vi "Stop Measurement.vi"(1 "VISA resource name":refnum<visa-resource-name>="COM1", 2 "Addr (0-15)":i8 min=0 max=15 step=1) -> (0 "Stop OK":bool)   [LabVIEW 2012]
doc: "The Basic Serial Read and Write example performs a Serial Port Read, a Serial Port Write, or a combination of these actions. The user selects the actions (read or write) on the front panel. If both are selected, the VI will write the data first, read data, and then close the VISA session that is opened to the port. This VI will wait until the specified number of bytes is received at the port or until a termination character is read.\n\nINSTRUCTIONS:\n1) Select the serial resource and configuration parameters (baud rate, data bits, parity, stop bits, flow control).\n2) Select the operations to be performed. \n3) Connect the serial port to your device. If no device is available, perform a loopback test by doing one of the following. Short pins 2 and 3 on a RS-232 cable or short pin 4 to pin 8 and pin 5 to pin 9 on a RS-485/422 cable. \n4) Run the VI to see the data read. (The \"read string\" will match the \"string to write\" if a loopback test was performed.)\n\nNote: The parameters set for the serial port must match the parameters of the connected instrument or device. In this example, the bytes to read parameter specifies the number of bytes that the serial port reads. If there were more bytes at the port than the number specified in bytes to read, those bytes would not be read. Also, if you specify to read more bytes than the number of bytes actually read, you might receive a timeout error message.\n\nOn the block diagram, the Configure Serial Port VI sets the configuration parameters. The front panel displays the controls used to configure the basic parameters, such as baud rate, data bits, and parity. Constants configure the other parameters the user probably does not need set. After the VISA Configure Serial Port VI opens the VISA session and configures the port, the VI passes the VISA resource name to other VIs that perform operations on that VISA resource. The VISA Write function sends a command to the serial device and the VISA Read function returns data based on the command. The VISA Close function then closes the reference to the serial device. It is important to close the reference; otherwise communication through with that port through protocols other than VISA might not be possible."
uses:
  <vilib>/Instr/_visa.llb/VISA Configure Serial Port (Instr).vi
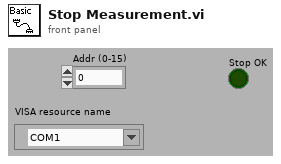
[diagram p1: front panel]
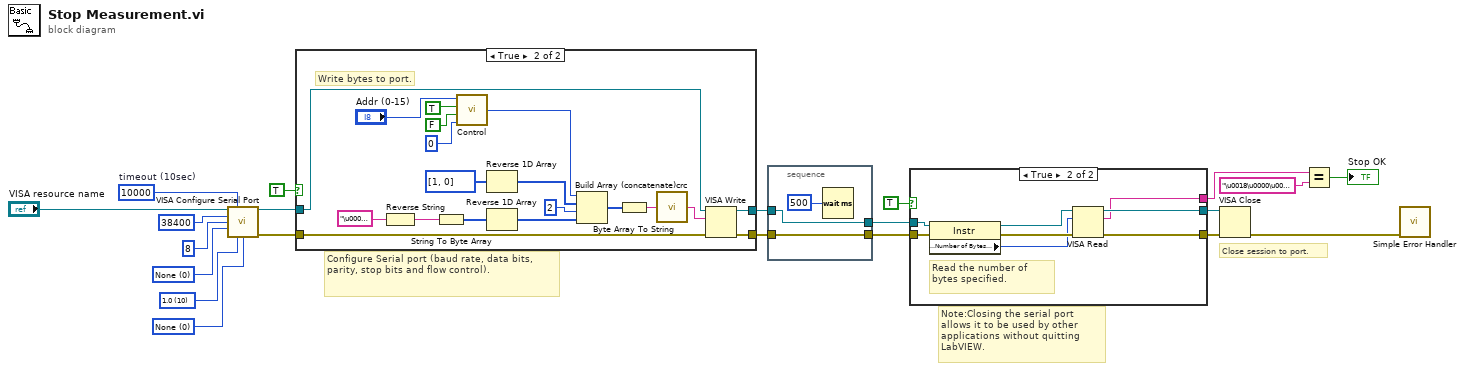
[diagram p0: block diagram]
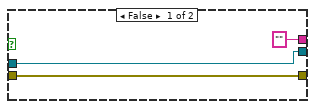
[diagram p3: hidden frame]
diagram:
  w11 = u16 0 items=["None"=0, "XON/XOFF"=1, "RTS/CTS"=2, "DTR/DSR"=4] ("flow control")
  w12 = u16 10 items=["1.0"=10, "1.5"=15, "2.0"=20] ("stop bits")
  w14 = u16 0 items=["None", "Odd", "Even", "Mark", "Space"] ("parity")
  w13 = u32 10000  # timeout (10sec)
  # "Note:Closing the serial port allows it to be used by other applications without quitting LabVIEW."
  # "Configure Serial port (baud rate, data bits, parity, stop bits and flow control)."
  # "Close session to port."
  n1 = call-poly "VISA Configure Serial Port"("VISA resource name"="VISA resource name", "timeout (10sec)"=w13, "baud rate (9600)"=u32 38400, "data bits (8)"=u16 8 ("data bits"), "parity (0:none)"=w14, "stop bits (10: 1 bit)"=w12, "flow control (0:none)"=w11) -> ("VISA resource name out"=w18:refnum<visa-resource-name>, "error out"=w19:errorcluster)  [unwired: 2 in, 5 out]
  n2 = case shown="True" TRUE ("write") {
    tunnel: [w23 w42] -> w8
    tunnel: w18 -> [w22 w41]
    tunnel: w19 -> [w23 w40]
    tunnel: [w22 w39] -> w6
    frame False {
    }
    frame True {
      # "Write bytes to port."
      n3 = Reverse String(1:"\u0000\u0000" ("Data")) -> (0:w24:string)
      n4 = String To Byte Array(string=w24) -> (unsigned byte array=w29:u8[])
      n5 = call "Control.vi"("Page"=i8 0, "Error"=FALSE, "Write"=TRUE, "Addr"="Addr (0-15)") -> ("Control Byte"=w34:u32)
      n6 = Reverse 1D Array(array=i8[] [1, 0] ("Offset")) -> (reversed array=w32:i8[])
      n7 = Reverse 1D Array(array=w29) -> (reversed array=w28:u8[])
      n8 = Build Array (concatenate)(w34, w32, u8 2 ("Length"), w28) -> (w27:u32[])
      n9 = Byte Array To String(unsigned byte array=w27) -> (string=w26:string)
      n10 = call "crc.vi"("Input string"=w26) -> ("Output (with crc)"=w25:string)
      n11 = VISA Write(VISA resource name=w41, write buffer=w25, error in (no error)=w40) -> (VISA resource name out=w39:refnum<visa-resource-name>, error out=w42:errorcluster)  [unwired: 1 out]
    }
  }
  n12 = stacked-sequence {
    tunnel: w8 -> [w45]
    tunnel: [w45] -> w7
    tunnel: w6 -> [w44]
    tunnel: [w44] -> w5
    frame #0 {
      n13 = Wait (ms)(milliseconds to wait=u32 500 ("delay before read (ms)")) -> ()  [unwired: 1 out]
    }
  }
  n14 = case shown="True" TRUE ("read") {
    tunnel: w7 -> [w48 w52]
    tunnel: [w48 w56] -> w17
    tunnel: [w47 w55] -> w16
    tunnel: w5 -> [w47 w54]
    tunnel: ["" ("read buffer") w49] -> w3
    frame False {
    }
    frame True {
      # "Read the number of bytes specified."
      n15 = property class="Instr"(reference=w54, error in=w52) -> (reference out=w53:refnum<visa-resource-name>, error out=w51:errorcluster, "Serial Settings:Number of Bytes at Serial Port"=w50:u32)
      n16 = VISA Read(VISA resource name=w53, byte count=w50, error in (no error)=w51) -> (VISA resource name out=w55:refnum<visa-resource-name>, read buffer=w49:string, error out=w56:errorcluster)  [unwired: 1 out]
    }
  }
  n17 = VISA Close(VISA resource name=w16, error in (no error)=w17) -> (error out=w15:errorcluster)
  n18 = Equal?(x=w3, y="\u0018\u0000\u0001\u0002Ì") -> (x = y?=→"Stop OK":bool)
  n19 = call <vilib>:"Simple Error Handler.vi"("error in (no error)"=w15) -> ()  [unwired: 1 in, 8 out]
